vi "BuildGraph.vi"(1 "X":dbl[](array[numeric]), 2 "Y":dbl[][](array[numeric])) -> (0 "Graph":cluster{"X":dbl[], "Y":dbl[]}[](array[cluster]))   [LabVIEW 2013]
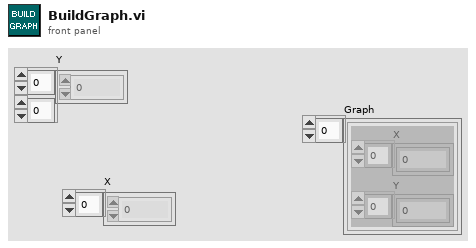
[diagram p1: front panel]
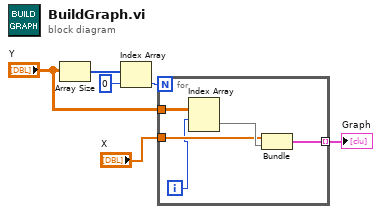
[diagram p0: block diagram]
diagram:
  n1 = Array Size(array="Y") -> (size(s)=w6:i32[])
  n2 = Index Array(array=w6, index=0) -> (element=w4:i32)
  n3 = for {
    N: w4 -> [_]
    tunnel: "Y" -> [w11]
    tunnel: "X" -> [w9]
    tunnel: [w8] -> w1 mode=indexing
    i -> [w7]
    n4 = Index Array(array=w11, index (row)=w7) -> (element=w10:dbl[])  [unwired: 1 in]
    n5 = Bundle("X"=w9, "Y"=w10) -> (w8:cluster{"X":dbl[], "Y":dbl[]})  [unwired: 1 in]
  }
  "Graph" <- w1
